vi "AO_formula.vi"() -> ()   [LabVIEW 2021]
uses:
  <vilib>/userdefined/High Color/nirio_resource_hc.ctl
  <vilib>/rvi/Analysis/host/Private/Sample Rate To Loop Time (ticks).vi
  <vilib>/FPGAPlugInAG/PCIe-7857/niLvFpga_Open_PCIe-7857.vi
  <vilib>/Utility/error.llb/Error Cluster From Error Code.vi
  <vilib>/rvi/errors/niLvFpgaAdjustHostInterfaceError.vi
  <vilib>/rvi/interface/common/niFpgaWaitOnOcc.vi
  <vilib>/FPGAPlugInAG/PCIe-7857/niLvFpga_Run_PCIe-7857.vi
  <vilib>/FPGAPlugInAG/PCIe-7857/niLvFpga_Close_PCIe-7857.vi
  <vilib>/rvi/interface/nirviOpenFPGA/nirviOpenFPGA.xnode
  FPGA Bitfiles/lvfpga2_FPGATarget_FPGA_J9MBVCOB9rw.lvbitx
  FPGA.vi
  <vilib>/rvi/interface/nirviReadWriteControl/nirviReadWriteControl.xnode
  <vilib>/rvi/interface/nirviMethod/nirviMethod.xnode
  <vilib>/rvi/interface/nirviCloseFPGA/nirviCloseFPGA.xnode
  <vilib>/rvi/errors/niLvFpgaMergeErrorWithErrorCode.vi
  <vilib>/FPGAPlugInAG/PCIe-7857/niLvFpga_WriteFifo_PCIe-7857.vi
  <vilib>/rvi/Analysis/host/Public/NI_FpgaMspHost.lvlib
  NiFpgaLv.dll
  <vilib>/FPGAPlugInAG/PCIe-7857/niLvFpga_ConfigureFifo_PCIe-7857.vi
panel:
  out "Actual #s":dbl
  in  "Signal Parameters":cluster{"Fs":dbl, "#s":dbl}={"Fs"=200000.0, "#s"=100.0} {"Fs" format="%#_6p"}
  out "dt":dbl
  in  "scale":sgl=1.0 format="%0.2f"
  in  "offset":sgl format="%0.2p"
  in  "functionInfo":T1={"time1"=5e-05, "formula1"="2", "time2"=5e-05, "formula2"="3", "time3"=0.0005, "formula3"="4", "time4"=0.001, "formula4"="1"}
  out "Actual Depth":u32
  out "Waveform Graph 2":dbl[](graph)
  out "Waveform Graph":waveform(dbl)(graph)
  in  "RIO Resource Name":T2="RIO0" caption="RIO Device"
  in  "stop":bool
  out "Actual Sample Clock Rate":dbl=20000.0 format="%.2f"
  # "实际点数为定义总时间乘以速率Fs，如果定义总时间小于信号点数，则为未定义时间赋0"
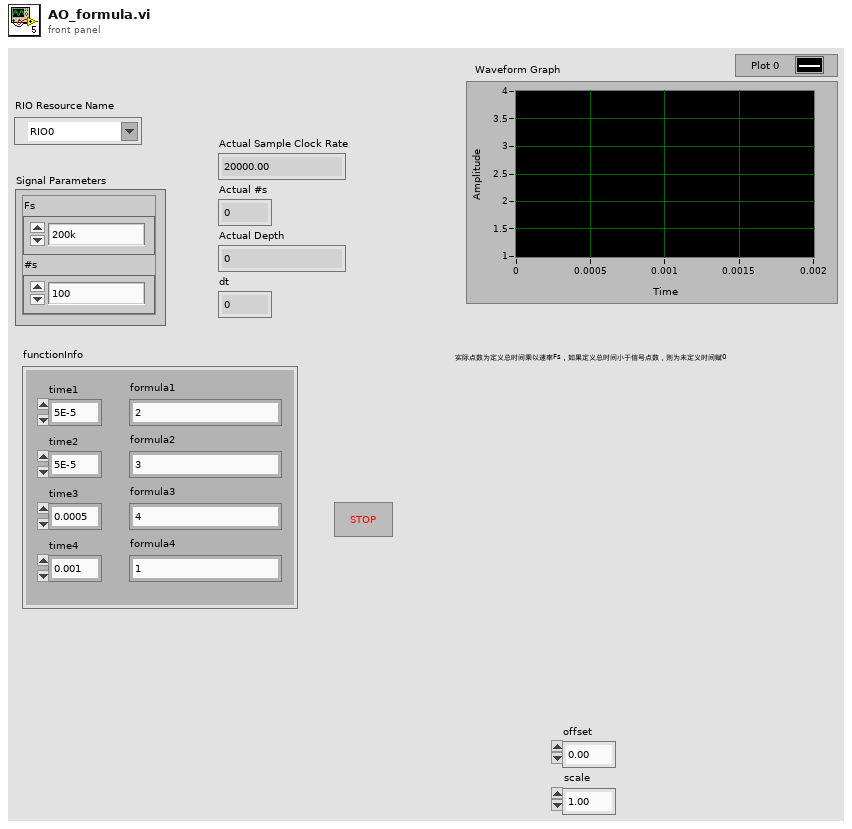
[diagram p1: front panel]
types:
  T1 = cluster{"time1":dbl, "formula1":string, "time2":dbl, "formula2":string, "time3":dbl, "formula3":string, "time4":dbl, "formula4":string}
  T2 = typedef "nirio_resource_hc.ctl" = tag
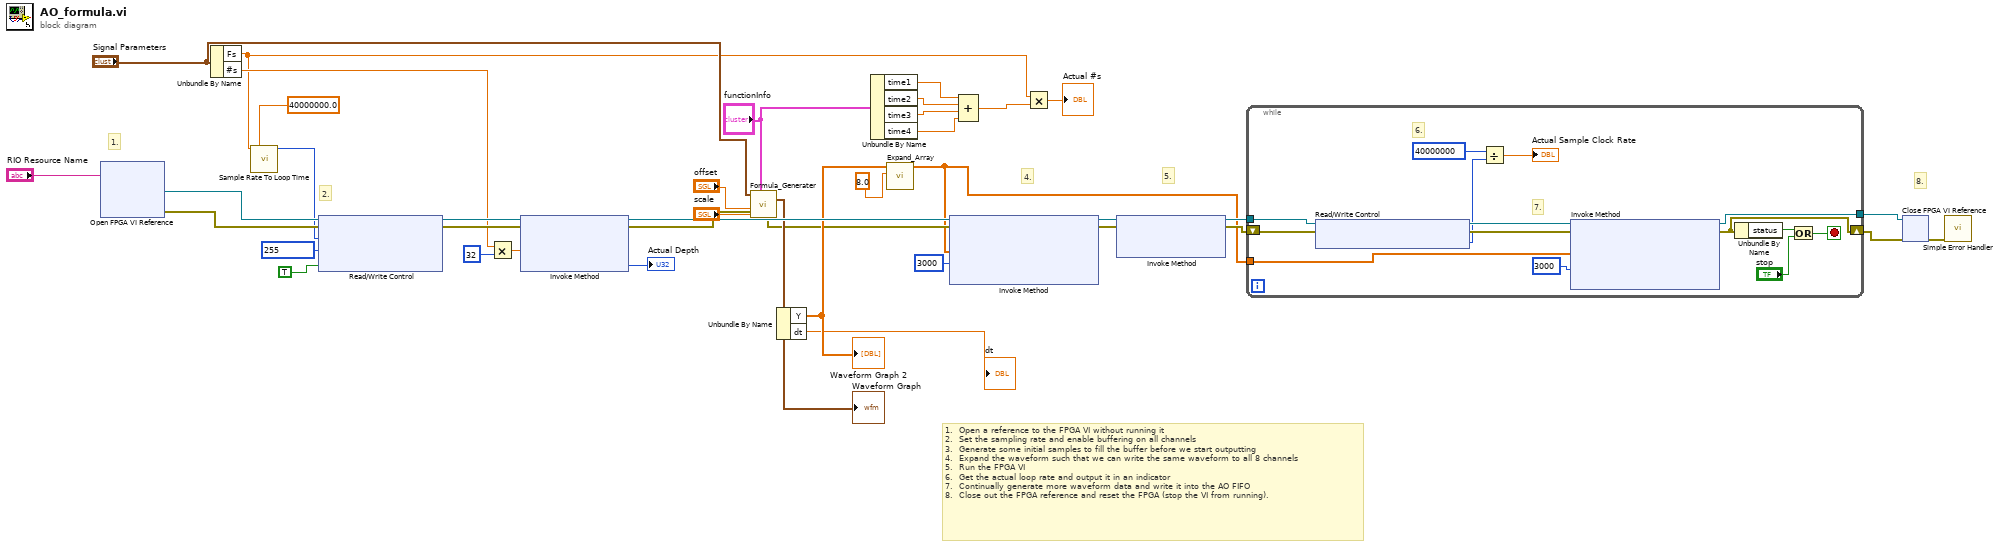
[diagram p0: block diagram]
diagram:
  # "1."
  # "1.  Open a reference to the FPGA VI without running it\n2.  Set the sampling rate and enable buffering on all channels\n3.  Generate some initial samples to fill the buffer before we start outputting\n4.  Expand the waveform such that we can write the same waveform to all 8 channels\n5.  Run the FPGA VI\n6.  Get the actual loop rate and output it in an indicator\n7.  Continually generate more waveform data and write it into the AO FIFO\n8.  Close out the FPGA reference and reset the FPGA (stop the VI from running)."
  # "8."
  # "5."
  # "4."
  # "2."
  n1 = xnode "Open FPGA VI Reference"("resource name"="RIO Resource Name") -> ("FPGA VI Reference Out"=w24:refnum<k20>, "error out"=w25:errorcluster)  [unwired: 1 in]
  n2 = Unbundle By Name("Signal Parameters") -> ("Fs"=w2:dbl, "#s"=w5:dbl)
  n3 = call-poly <vilib>:"Sample Rate To Loop Time.vi"("sample rate (S/s)"=w2, "FPGA clock rate (Hz)"=40000000.0) -> ("count (ticks/S)"=w7:u32)  [unwired: 11 in, 2 out]
  n4 = xnode "Read/Write Control"("FPGA VI Reference In"=w24, "error in"=w25, "AO Loop Timer (ticks)"=w7, "AO Buffer Enable"=u8 255, "AO Enable"=TRUE) -> ("FPGA VI Reference Out"=w31:refnum<k20>, "error out"=w30:errorcluster)
  n5 = Multiply(x=w5, y=u32 32) -> (x*y=w27:dbl)
  n6 = xnode "Invoke Method"("FPGA VI Reference In"=w31, "error in"=w30, "Requested Depth"=w27) -> ("FPGA VI Reference Out"=w29:refnum<k20>, "error out"=w18:errorcluster, "Actual Depth"=→"Actual Depth":u32)
  n7 = call "Formula_Generater.vi"("error in (no error)"=w18, "functionInfo"="functionInfo", "scale"="scale", "offset"="offset", "sampling info"="Signal Parameters") -> ("error out"=w17:errorcluster, "waveform out"=w20:waveform(dbl))  [unwired: 5 in]
  "Waveform Graph" <- w20
  n8 = Unbundle By Name(w20) -> ("Y"=w21:dbl[], "dt"=→"dt":dbl)
  "Waveform Graph 2" <- w21
  n9 = Unbundle By Name("functionInfo") -> ("time1"=w12:dbl, "time2"=w11:dbl, "time3"=w10:dbl, "time4"=w9:dbl)
  n10 = call "Expand_Array.vi"("Scale Factor"=sgl 8.0, "Input AO Array"=w21) -> ("Output Array"=w14:sgl[])  [unwired: 9 in]
  n11 = xnode "Invoke Method"("FPGA VI Reference In"=w29, "error in"=w17, "Data"=w14, "Timeout (ms)"=3000) -> ("FPGA VI Reference Out"=w19:refnum<k20>, "error out"=w32:errorcluster)  [unwired: 1 out]
  n12 = Compound Arithmetic op=ADD(w12, w11, w10, w9) -> (w3:dbl)
  n13 = Multiply(x=w2, y=w3) -> (x*y=→"Actual #s":dbl)
  n14 = xnode "Invoke Method"("FPGA VI Reference In"=w19, "error in"=w32) -> ("FPGA VI Reference Out"=w37:refnum<k20>, "error out"=w36:errorcluster)  [unwired: 1 in]
  n15 = while {
    tunnel: w37 -> [w52]
    shift-right: [w44] -> w34
    shift-left: w36 -> [w41]
    tunnel: [w54] -> w35
    tunnel: w14 -> [w42]
    stop <- w45 stop-if-true
    # "7."
    # "6."
    n16 = xnode "Read/Write Control"("FPGA VI Reference In"=w52, "error in"=w41) -> ("FPGA VI Reference Out"=w51:refnum<k20>, "error out"=w50:errorcluster, "AO: Actual Loop Rate (ticks)"=w49:u32)
    n17 = Divide(x=u32 40000000, y=w49) -> (x/y=→"Actual Sample Clock Rate":dbl)
    n18 = xnode "Invoke Method"("FPGA VI Reference In"=w51, "error in"=w50, "Data"=w42, "Timeout (ms)"=3000) -> ("FPGA VI Reference Out"=w54:refnum<k20>, "error out"=w44:errorcluster)  [unwired: 1 out]
    n19 = Unbundle By Name(w44) -> ("status"=w43:bool)
    n20 = Or(x=w43, y="stop") -> (x .or. y?=w45:bool)
  }
  n21 = xnode "Close FPGA VI Reference"("FPGA VI Reference In"=w35, "error in"=w34) -> ("error out"=w33:errorcluster)
  n22 = call <vilib>:"Simple Error Handler.vi"("error in (no error)"=w33) -> ()  [unwired: 4 in, 5 out]
